vi "DataSave.vi"(10 "Experiment State":T1={"Send Trigger 3"=FALSE, "error"={"status"=FALSE, "code"=0, "source"=""}, "Tasks"={"Fiber15 MP Task"="MyVoltageTask", "Read Slow AI"="", "Fiber Bank DIO"="", "Fiber7 MP Task"="MyVoltageTask", "TaskArray"=[]}, "Channels"={"6133 Channels"=[], "Edge Type"=10280, "Samples Per Channel"=[], "#Pre-Trigger Samples"=[], "Sample Rate 2.5Ms/s Max"=[], "Trigger Sources"=[], "Voltage Ranges"=[], "Channel Names"=[], "Active"=[]}, "Dev 10 DIO"="", "Dev5"="", "Fiber Triggers 2"=[{"Delay (s)"=2.559999942779541, "Pulse width (s)"=0.009999999776482582, "Active"=TRUE, "Channel Name"="Fiber 8", "counter"="PXI1Slot8/ctr7"}], "MP7"=FALSE, "MP15"=FALSE, "PXI Slot 2"={"PXI Slot 2 Handle"="PXI1Slot2", "source terminal"="GlobalSoftwareTrigger"}, "# of Control DIOs"=0, "Bank DIO Settings"=[], "Purge Duration (s)"=5, "Interlock Override"=FALSE, "Current Raw Voltages, Slot &"=[], "Bank Control"={"Bank Enables"={"Gun1 Enable"=FALSE, "Gun2 Enable"=FALSE, "InnerSol Enable"=FALSE, "OuterSol1 Enable"=FALSE, "Outer2 Enable"=FALSE, "Gun3 Enable"=FALSE}, "Voltages"={"Gun1 Voltage"=0.0, "Gun2 Voltage"=0.0, "Gun3 Voltage"=0.0, "InnerSol Voltage"=0.0, "OuterSol1 Voltage"=0.0, "OuterSol2 Voltage"=0.0}, "Set Points"={"Gun1 Setpoint"=0.0, "Gun2 Setpoint"=0.0, "Gun3 Setpoint"=0.0, "InnerSol Setpoint"=0.0, "OuterSol1 Setpoint"=0.0, "OuterSol2 Setpoint"=0.0}}, "Waveform Data"=[], "Next Shot#"="0", "Slot 7, Last Shot Scaled Voltages"=[], "Data Run Description"="", "Next Shot Data"=["599", "6/18/2009", "4:08PM", "Ziemba", "Bank Testing", "-7.142518", "-8.256295", "-6.893030", "-5.120022", "-0.001235", "-0.001559", "-0.000910", "-0.001235", "-0.001235", "-0.001235", "-0.001235", "0.114909", "-0.000586", "-0.000586", "0.684598", "1.197512"], "Headers"=[], "Html Shot Log View"=FALSE, "ShotLog Headers"=path "", "ShotLog Data"=path "", "Enable Bank Control"=FALSE, "6602  Slot8"={"Slot 8 Trigger Source"="", "Slot 8 Clock Source"="", "Trigger Channel Tasks"=[]}, "6602  Slot 9"={"Slot 9 Clock Source"="", "Slot 9 Trigger Source"="", "Trigger Channel Tasks"=[]}, "Total Sample Time (us)"=[], "Pre-Trigger Time (us)"=[], "Fiber Triggers"=[{"Delay (s)"=2.559999942779541, "Pulse width (s)"=0.009999999776482582, "Active"=TRUE, "Channel Name"="Fiber 8", "counter"="PXI1Slot8/ctr7"}], "System Message"=""} {"Fiber Triggers"."Pulse width (s)" format="%.3p"; "Fiber Triggers"."Delay (s)" format="%.3p"; "Pre-Trigger Time (us)" format="%#_6f"; "Total Sample Time (us)" format="%#_6f"; "Current Raw Voltages, Slot &" format="%0.2f"; "Fiber Triggers 2"."Pulse width (s)" format="%.3p"; "Fiber Triggers 2"."Delay (s)" format="%.3p"; "Channels"."Sample Rate 2.5Ms/s Max" format="%#_3p"; "Channels"."Edge Type" items=["Rising"=10280, "Falling"=10171]}, 11 "All Data":string[](array[string])) -> (2 "Experiment State":T1={"Send Trigger 3"=FALSE, "error"={"status"=FALSE, "code"=0, "source"=""}, "Tasks"={"Fiber15 MP Task"="MyVoltageTask", "Read Slow AI"="", "Fiber Bank DIO"="", "Fiber7 MP Task"="MyVoltageTask", "TaskArray"=[]}, "Channels"={"6133 Channels"=[], "Edge Type"=10280, "Samples Per Channel"=[], "#Pre-Trigger Samples"=[], "Sample Rate 2.5Ms/s Max"=[], "Trigger Sources"=[], "Voltage Ranges"=[], "Channel Names"=[], "Active"=[]}, "Dev 10 DIO"="", "Dev5"="", "Fiber Triggers 2"=[{"Delay (s)"=2.559999942779541, "Pulse width (s)"=0.009999999776482582, "Active"=TRUE, "Channel Name"="Fiber 8", "counter"="PXI1Slot8/ctr7"}], "MP7"=FALSE, "MP15"=FALSE, "PXI Slot 2"={"PXI Slot 2 Handle"="PXI1Slot2", "source terminal"="GlobalSoftwareTrigger"}, "# of Control DIOs"=0, "Bank DIO Settings"=[], "Purge Duration (s)"=5, "Interlock Override"=FALSE, "Current Raw Voltages, Slot &"=[], "Bank Control"={"Bank Enables"={"Gun1 Enable"=FALSE, "Gun2 Enable"=FALSE, "InnerSol Enable"=FALSE, "OuterSol1 Enable"=FALSE, "Outer2 Enable"=FALSE, "Gun3 Enable"=FALSE}, "Voltages"={"Gun1 Voltage"=0.0, "Gun2 Voltage"=0.0, "Gun3 Voltage"=0.0, "InnerSol Voltage"=0.0, "OuterSol1 Voltage"=0.0, "OuterSol2 Voltage"=0.0}, "Set Points"={"Gun1 Setpoint"=0.0, "Gun2 Setpoint"=0.0, "Gun3 Setpoint"=0.0, "InnerSol Setpoint"=0.0, "OuterSol1 Setpoint"=0.0, "OuterSol2 Setpoint"=0.0}}, "Waveform Data"=[], "Next Shot#"="0", "Slot 7, Last Shot Scaled Voltages"=[], "Data Run Description"="", "Next Shot Data"=["599", "6/18/2009", "4:08PM", "Ziemba", "Bank Testing", "-7.142518", "-8.256295", "-6.893030", "-5.120022", "-0.001235", "-0.001559", "-0.000910", "-0.001235", "-0.001235", "-0.001235", "-0.001235", "0.114909", "-0.000586", "-0.000586", "0.684598", "1.197512"], "Headers"=[], "Html Shot Log View"=FALSE, "ShotLog Headers"=path "", "ShotLog Data"=path "", "Enable Bank Control"=FALSE, "6602  Slot8"={"Slot 8 Trigger Source"="", "Slot 8 Clock Source"="", "Trigger Channel Tasks"=[]}, "6602  Slot 9"={"Slot 9 Clock Source"="", "Slot 9 Trigger Source"="", "Trigger Channel Tasks"=[]}, "Total Sample Time (us)"=[], "Pre-Trigger Time (us)"=[], "Fiber Triggers"=[{"Delay (s)"=2.559999942779541, "Pulse width (s)"=0.009999999776482582, "Active"=TRUE, "Channel Name"="Fiber 8", "counter"="PXI1Slot8/ctr7"}], "System Message"=""} {"Fiber Triggers"."Pulse width (s)" format="%.3p"; "Fiber Triggers"."Delay (s)" format="%.3p"; "Pre-Trigger Time (us)" format="%#_6f"; "Total Sample Time (us)" format="%#_6f"; "Current Raw Voltages, Slot &" format="%0.2f"; "Fiber Triggers 2"."Pulse width (s)" format="%.3p"; "Fiber Triggers 2"."Delay (s)" format="%.3p"; "Channels"."Sample Rate 2.5Ms/s Max" format="%#_3p"; "Channels"."Edge Type" items=["Rising"=10280, "Falling"=10171]}, 3 "Data Save Results":T2)   [LabVIEW 2013]
uses:
  Controls/ExperimentStateCluster.ctl
  <vilib>/Waveform/WDTFileIO.llb/Export Waveforms To Spreadsheet File (2D).vi
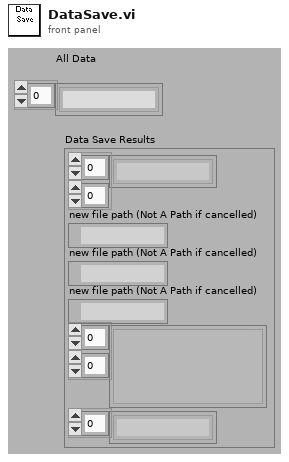
[diagram p1: front panel]
types:
  T1 = typedef "ExperimentStateCluster.ctl" = cluster{"Send Trigger 3":bool, "error":errorcluster, "Tasks":cluster{"Fiber15 MP Task":refnum<k21>, "Read Slow AI":refnum<k21>, "Fiber Bank DIO":refnum<k21>, "Fiber7 MP Task":refnum<k21>, "TaskArray":refnum<k21>[]}, "Channels":cluster{"6133 Channels":tag[][], "Edge Type":i32, "Samples Per Channel":i32[], "#Pre-Trigger Samples":u32[], "Sample Rate 2.5Ms/s Max":dbl[], "Trigger Sources":tag[], "Voltage Ranges":dbl[][], "Channel Names":string[][], "Active":bool[][]}, "Dev 10 DIO":refnum<k21>, "Dev5":refnum<k21>, "Fiber Triggers 2":cluster{"Delay (s)":dbl, "Pulse width (s)":dbl, "Active":bool, "Channel Name":string, "counter":tag}[], "MP7":bool, "MP15":bool, "PXI Slot 2":cluster{"PXI Slot 2 Handle":refnum<k15>, "source terminal":string}, "# of Control DIOs":i32, "Bank DIO Settings":bool[], "Purge Duration (s)":u32, "Interlock Override":bool, "Current Raw Voltages, Slot &":dbl[], "Bank Control":cluster{"Bank Enables":cluster{"Gun1 Enable":bool, "Gun2 Enable":bool, "InnerSol Enable":bool, "OuterSol1 Enable":bool, "Outer2 Enable":bool, "Gun3 Enable":bool}, "Voltages":cluster{"Gun1 Voltage":dbl, "Gun2 Voltage":dbl, "Gun3 Voltage":dbl, "InnerSol Voltage":dbl, "OuterSol1 Voltage":dbl, "OuterSol2 Voltage":dbl}, "Set Points":cluster{"Gun1 Setpoint":dbl, "Gun2 Setpoint":dbl, "Gun3 Setpoint":dbl, "InnerSol Setpoint":dbl, "OuterSol1 Setpoint":dbl, "OuterSol2 Setpoint":dbl}}, "Waveform Data":waveform(dbl)[][], "Next Shot#":string, "Slot 7, Last Shot Scaled Voltages":string[], "Data Run Description":string, "Next Shot Data":string[], "Headers":string[], "Html Shot Log View":bool, "ShotLog Headers":path, "ShotLog Data":path, "Enable Bank Control":bool, "6602  Slot8":cluster{"Slot 8 Trigger Source":tag, "Slot 8 Clock Source":tag, "Trigger Channel Tasks":refnum<k21>[]}, "6602  Slot 9":cluster{"Slot 9 Clock Source":tag, "Slot 9 Trigger Source":tag, "Trigger Channel Tasks":refnum<k21>[]}, "Total Sample Time (us)":dbl[], "Pre-Trigger Time (us)":dbl[], "Fiber Triggers":cluster{"Delay (s)":dbl, "Pulse width (s)":dbl, "Active":bool, "Channel Name":string, "counter":tag}[], "System Message":string}
  T2 = cluster{string[][], "new file path (Not A Path if cancelled)":path, "new file path (Not A Path if cancelled)":path, "new file path (Not A Path if cancelled)":path, variant[][], string[]}
  T3 = cluster{"Delay (s)":dbl, "Pulse width (s)":dbl, "Active":bool, "Channel Name":string, "counter":tag}[]
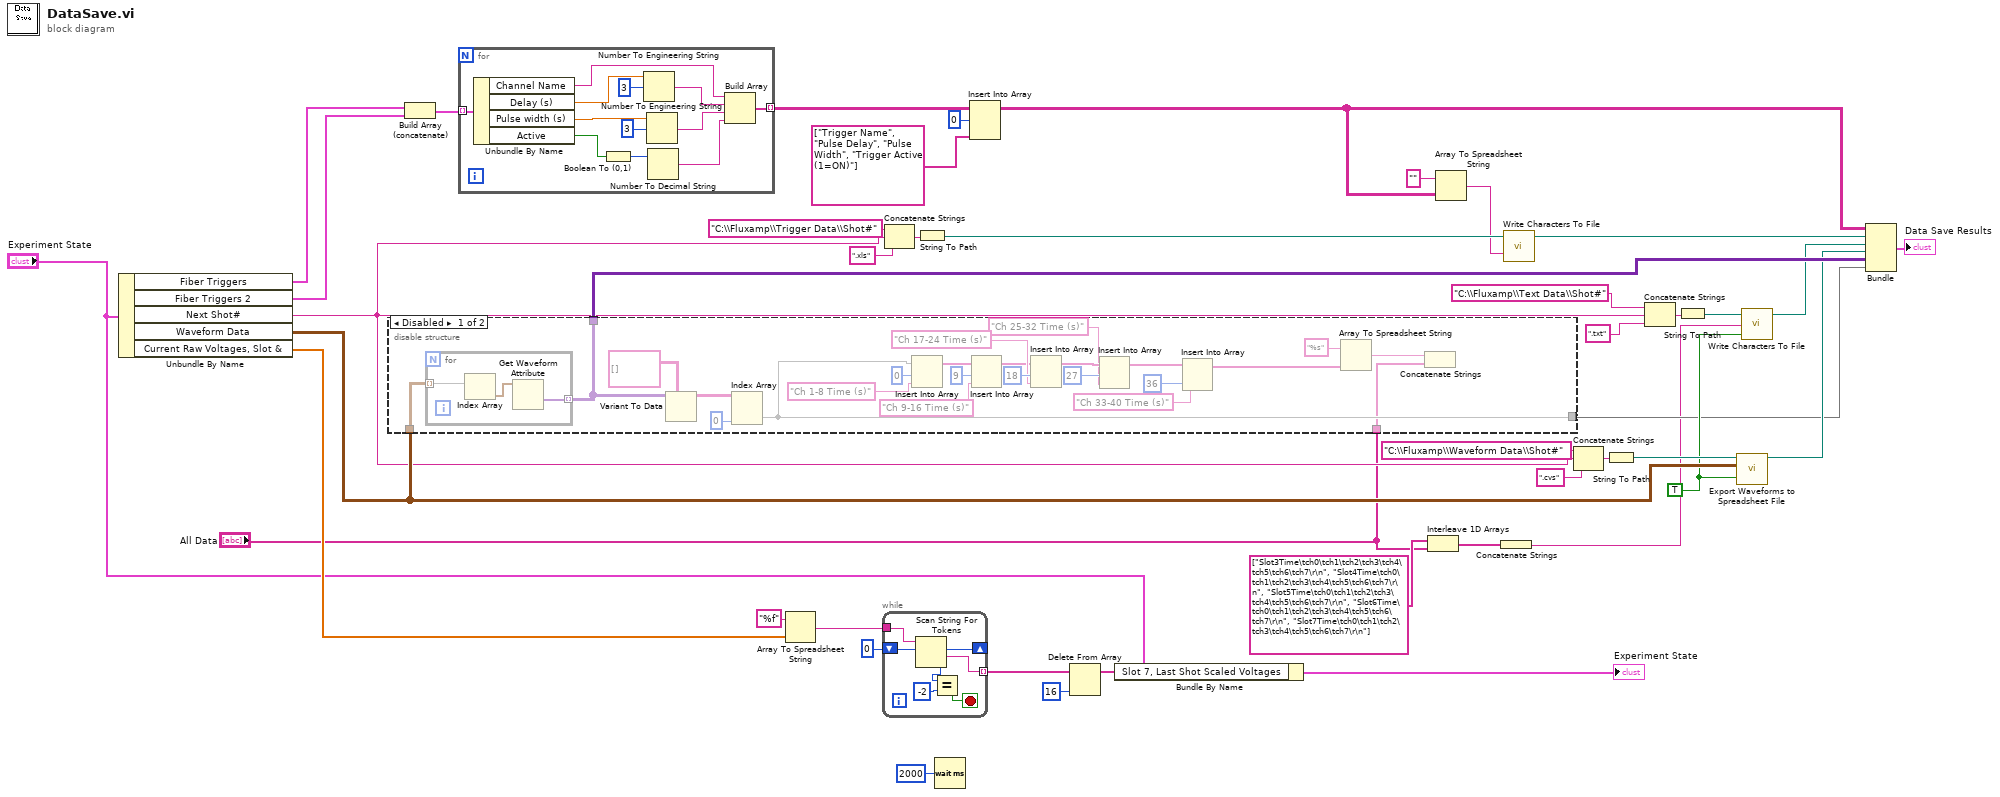
[diagram p0: block diagram]
diagram:
  w6 = TRUE ("append to file? (new file:F)")
  n1 = Unbundle By Name("Experiment State") -> ("Fiber Triggers"=w36:T3, "Fiber Triggers 2"=w37:T3, "Next Shot#"=w28:string, "Waveform Data"=w29:waveform(dbl)[][], "Current Raw Voltages, Slot &"=w38:dbl[])
  n2 = disable-structure shown="Disabled" {
    disable-tunnel: [w68 _] -> w44
    disable-tunnel: w29 -> [w67 _]
    disable-tunnel: [w46 _] -> w5
    disable-tunnel: "All Data" -> [w45 _]
    frame Disabled {
      n3 = for {
        tunnel: w67 -> [w70] mode=indexing
        tunnel: [w71] -> w68 mode=indexing
        n4 = Index Array(array=w70) -> (element=w69:waveform(dbl))  [unwired: 1 in]
        n5 = Get Waveform Attribute(7:w69) -> (1:w71:variant[])  [unwired: 1 in, 5 out]
      }
      n6 = Variant To Data(type=string[][] [], Variant=w68) -> (data=w65:string[][])  [unwired: 1 in, 1 out]
      n7 = Index Array(array=w65, index (col)=0 ("disabled index (col)")) -> (element=w46:string[])  [unwired: 1 in]
      n8 = Insert Into Array(array=w46, index=0, new element="Ch 1-8 Time (s)" ("new element/subarray")) -> (w61:string[])
      n9 = Insert Into Array(array=w61, index=9, new element="Ch 9-16 Time (s)" ("new element/subarray")) -> (w51:string[])
      n10 = Insert Into Array(array=w51, index=18, new element="Ch 17-24 Time (s)" ("new element/subarray")) -> (w54:string[])
      n11 = Insert Into Array(array=w54, index=27, new element="Ch 25-32 Time (s)" ("new element/subarray")) -> (w49:string[])
      n12 = Insert Into Array(array=w49, index=36, new element="Ch 33-40 Time (s)" ("new element/subarray")) -> (w47:string[])
      n13 = Array To Spreadsheet String(array=w47, 3:"%s" ("format string")) -> (spreadsheet string=w58:string)  [unwired: 1 out]
      n14 = Concatenate Strings(w58, w45) -> ()  [unwired: 1 out]
    }
    frame Enabled {
    }
  }
  n15 = Build Array (concatenate)(w36, w37) -> (w10:T3)
  n16 = for {
    tunnel: w10 -> [w83] mode=indexing
    tunnel: [w73] -> w9 mode=indexing
    n17 = Unbundle By Name(w83) -> ("Channel Name"=w72:string, "Delay (s)"=w82:dbl, "Pulse width (s)"=w79:dbl, "Active"=w76:bool)
    n18 = Boolean To (0,1)(Boolean=w76) -> (0, 1=w75:i16)
    n19 = Number To Engineering String(3:i16 3 ("width (-)"), 4:w82) -> (0:w77:string)  [unwired: 2 out]
    n20 = Number To Engineering String(3:i16 3 ("width (-)"), 4:w79) -> (0:w78:string)  [unwired: 2 out]
    n21 = Number To Decimal String(number=w75) -> (decimal integer string=w74:string)  [unwired: 1 out]
    n22 = Build Array(w72, w77, w78, w74) -> (w73:string[])
  }
  n23 = Array To Spreadsheet String(array=w38, 3:"%f" ("format string")) -> (spreadsheet string=w32:string)  [unwired: 1 out]
  n24 = while {
    tunnel: w32 -> [w90]
    shift-right: [w88] -> _
    shift-left: 0 ("offset past token") -> [w89]
    tunnel: [w84] -> w34 mode=indexing
    stop <- w85 stop-if-true
    n25 = Scan String For Tokens(8:w89, 9:w90) -> (0:w87:i32, 1:w84:string, 2:w88:i32)  [unwired: 5 out]
    n26 = Equal?(x=w87, y=-2) -> (x = y?=w85:bool)
  }
  n27 = Concatenate Strings("C:\\Fluxamp\\Trigger Data\\Shot#" ("string"), w28, ".xls" ("string")) -> (w15:string)
  n28 = String To Path(string=w15) -> (path=w14:path)
  n29 = Wait (ms)(milliseconds to wait=u32 2000) -> ()  [unwired: 1 out]
  n30 = Insert Into Array(array=w9, index (row)=0, new element=string[] ["Trigger Name", "Pulse Delay", "Pulse Width", "Trigger Active (1=ON)"] ("new element/subarray")) -> (w40:string[][])  [unwired: 1 in]
  n31 = Delete From Array(array=w34, index=16) -> (array with subset deleted=w39:string[])  [unwired: 1 in, 1 out]
  n32 = Bundle By Name(cluster="Experiment State", "Slot 7, Last Shot Scaled Voltages"=w39) -> (→"Experiment State":T1)
  n33 = Interleave 1D Arrays(string[] ["Slot3Time\tch0\tch1\tch2\tch3\tch4\tch5\tch6\tch7\r\n", "Slot4Time\tch0\tch1\tch2\tch3\tch4\tch5\tch6\tch7\r\n", "Slot5Time\tch0\tch1\tch2\tch3\tch4\tch5\tch6\tch7\r\n", "Slot6Time\tch0\tch1\tch2\tch3\tch4\tch5\tch6\tch7\r\n", "Slot7Time\tch0\tch1\tch2\tch3\tch4\tch5\tch6\tch7\r\n"], "All Data") -> (w4:string[])
  n34 = Array To Spreadsheet String(array=w40, 3:"" ("format string")) -> (spreadsheet string=w7:string)  [unwired: 1 in]
  n35 = Concatenate Strings(w4) -> (w3:string)
  n36 = call <vilib>:"Write Characters To File.vi"("character string"=w7, "file path (dialog if empty)"=w14) -> ("new file path (Not A Path if cancelled)"=w41:path)  [unwired: 1 in, 2 out]
  n37 = Concatenate Strings("C:\\Fluxamp\\Waveform Data\\Shot#" ("string"), w28, ".cvs" ("string")) -> (w19:string)
  n38 = String To Path(string=w19) -> (path=w18:path)
  n39 = Concatenate Strings("C:\\Fluxamp\\Text Data\\Shot#" ("string"), w28, ".txt" ("string")) -> (w22:string)
  n40 = String To Path(string=w22) -> (path=w11:path)
  n41 = call-poly <vilib>:"Export Waveforms to Spreadsheet File.vi"("append to file? (new file:F)"=w6, "waveforms"=w29, "file path (dialog if empty)"=w18) -> ("new file path (Not A Path if cancelled)"=w43:path)  [unwired: 7 in, 1 out]
  n42 = call <vilib>:"Write Characters To File.vi"("append to file? (new file:F)"=w6, "character string"=w3, "file path (dialog if empty)"=w11) -> ("new file path (Not A Path if cancelled)"=w42:path)  [unwired: 2 out]
  n43 = Bundle(w40, "new file path (Not A Path if cancelled)"=w41, "new file path (Not A Path if cancelled)"=w42, "new file path (Not A Path if cancelled)"=w43, w44, w5) -> (→"Data Save Results":T2)  [unwired: 1 out]
